vi "Global Offset Creator.vi"(4 "Width Offset":u64, 5 "Height Offset":u64, 6 "Depth Offset":u64, 7 "Dimension":T1 {"Width" min=1; "Height" min=1; "Depth" min=1}) -> (0 "Thread Dimensions":T1={"Depth"=1, "Height"=1, "Width"=1} {"Width" min=1; "Height" min=1; "Depth" min=1}, 1 "Global Offset":T1 {"Width" min=1; "Height" min=1; "Depth" min=1})   [LabVIEW 2012]
doc: "This is a convenience VI that is used to automatically compute and provide Global Thread Offset and Global Threads based on input dimensions and Depth, Width, and Height.\n\nFor example, if the number of threads is 1, 512, 980 (D, W, H) and the algorithm uses an offset of 4, 4, 4 (D, W, H), the Global Offset is 4, 4, 4 (D, W, H) and the Global Threads is now 1, 504, 972 (D, W, H)."
uses:
  User Controls/Array Dimensions.ctl
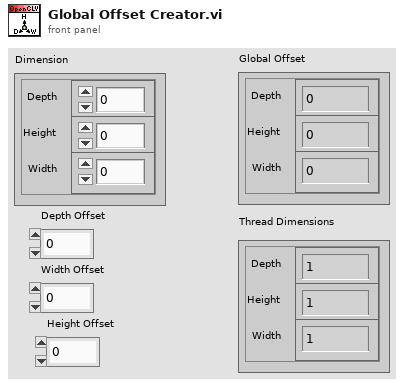
[diagram p1: front panel]
types:
  T1 = typedef "Array Dimensions.ctl" = cluster{"Depth":u64, "Height":u64, "Width":u64}
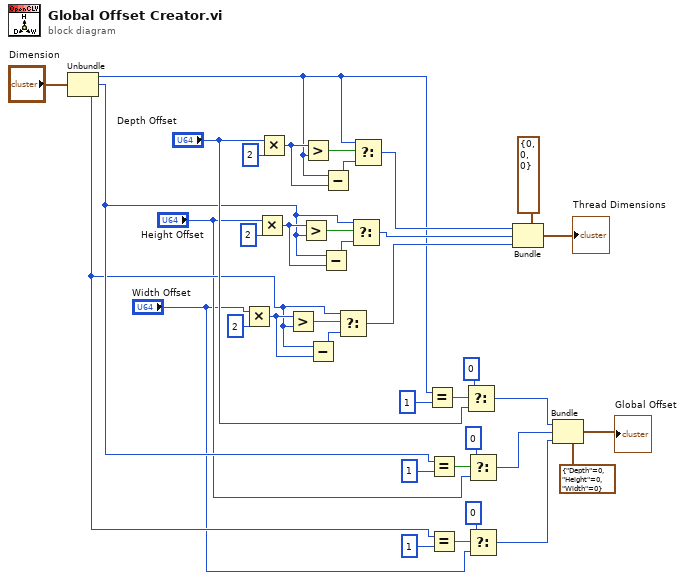
[diagram p0: block diagram]
diagram:
  n1 = Unbundle("Dimension") -> ("Depth"=w17:u64, "Height"=w4:u64, "Width"=w3:u64)
  n2 = Multiply(x="Width Offset", y=u64 2) -> (x*y=w25:u64)
  n3 = Multiply(x="Height Offset", y=u64 2) -> (x*y=w30:u64)
  n4 = Multiply(x="Depth Offset", y=u64 2) -> (x*y=w33:u64)
  n5 = Greater?(x=w25, y=w3) -> (0:w26:bool)
  n6 = Greater?(x=w30, y=w4) -> (0:w29:bool)
  n7 = Greater?(x=w33, y=w17) -> (0:w34:bool)
  n8 = Subtract(x=w3, y=w25) -> (x-y=w24:u64)
  n9 = Subtract(x=w4, y=w30) -> (x-y=w31:u64)
  n10 = Subtract(x=w17, y=w33) -> (x-y=w32:u64)
  n11 = Select(t=w3, s=w26, f=w24) -> (s? t:f=w21:u64)
  n12 = Select(t=w4, s=w29, f=w31) -> (s? t:f=w22:u64)
  n13 = Select(t=w17, s=w34, f=w32) -> (s? t:f=w23:u64)
  n14 = Equal?(x=w17, y=u64 1) -> (x = y?=w18:bool)
  n15 = Equal?(x=w4, y=u64 1) -> (x = y?=w10:bool)
  n16 = Equal?(x=w3, y=u64 1) -> (x = y?=w9:bool)
  n17 = Select(t=u64 0, s=w18, f="Depth Offset") -> (s? t:f=w13:u64)
  n18 = Select(t=u64 0, s=w10, f="Height Offset") -> (s? t:f=w6:u64)
  n19 = Select(t=u64 0, s=w9, f="Width Offset") -> (s? t:f=w5:u64)
  n20 = Bundle(cluster=cluster{"Depth":u64, "Height":u64, "Width":u64} {"Depth"=0, "Height"=0, "Width"=0} ("output cluster"), "Depth"=w23, "Height"=w22, "Width"=w21) -> (→"Thread Dimensions":cluster{"Depth":u64, "Height":u64, "Width":u64})
  n21 = Bundle(cluster=T1 {"Depth"=0, "Height"=0, "Width"=0} ("Global Offset"), "Depth"=w13, "Height"=w6, "Width"=w5) -> (→"Global Offset":T1)
